vi "Test Relays.vi"(8 "error in (no error)":errorcluster, 9 "relays":T1, 10 "state":u16(ring) items=["off", "on"], 11 "VGC in":refnum<class "PL Inficon VGC.lvclass">) -> (0 "error out":errorcluster, 1 "relays":T1, 2 "state":u16(ring) items=["off", "on"], 3 "VGC out":refnum<class "PL Inficon VGC.lvclass">)   [LabVIEW 2015, in "PL Inficon VGC.lvclass"]
doc: "Tests relays."
uses:
  PL Inficon VGC.lvclass
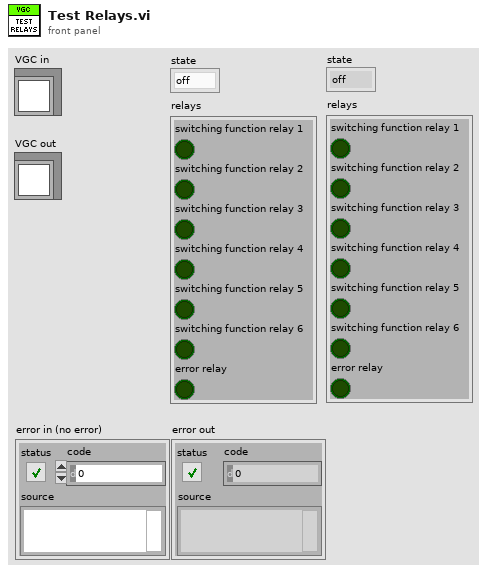
[diagram p1: front panel]
types:
  T1 = cluster{"switching function relay 1":bool, "switching function relay 2":bool, "switching function relay 3":bool, "switching function relay 4":bool, "switching function relay 5":bool, "switching function relay 6":bool, "error relay":bool}
  T2 = cluster{"Boolean array[0]":bool, "Boolean array[1]":bool, "Boolean array[2]":bool, "Boolean array[3]":bool, "Boolean array[4]":bool, "Boolean array[5]":bool, "Boolean array[6]":bool}
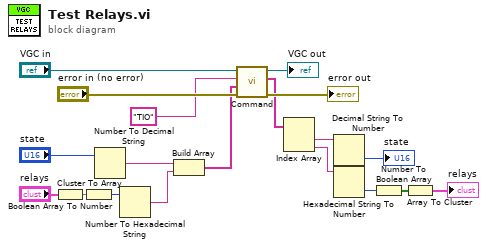
[diagram p0: block diagram]
diagram:
  n1 = Cluster To Array(cluster="relays") -> (array=w13:bool[])
  n2 = Boolean Array To Number(Boolean array=w13) -> (number=w4:u32)
  n3 = Number To Decimal String(number="state") -> (decimal integer string=w9:string)  [unwired: 1 in]
  n4 = Number To Hexadecimal String(2:w4) -> (0:w1:string)  [unwired: 1 in]
  n5 = Build Array(w9, w1) -> (w8:string[])
  n6 = call "Command.vi"("error in (no error)"="error in (no error)", "parameters"=w8, "command"="TIO", "VGC in"="VGC in") -> ("error out"=→"error out":errorcluster, "response data"=w7:string[], "VGC out"=→"VGC out":refnum<class "PL Inficon VGC.lvclass">)  [unwired: 5 in]
  n7 = Index Array(array=w7) -> (element #1=w6:string, element #2=w3:string)  [unwired: 2 in]
  n8 = Decimal String To Number(string=w6) -> (number=→"state":i32)  [unwired: 2 in, 1 out]
  n9 = Hexadecimal String To Number(string=w3) -> (number=w2:u32)  [unwired: 2 in, 1 out]
  n10 = Number To Boolean Array(number=w2) -> (Boolean array=w12:bool[])
  n11 = Array To Cluster(array=w12) -> (cluster=→"relays":T2)
